vi "MGI Set Z Scale Colors.vi"(7 "Scheme":T1=enum."Color Normal", 8 "error in (no error)":errorcluster, 9 "Min":dbl, 10 "Max":dbl, 11 "Scale or Intensity Graph Ref":refnum<vi>) -> (0 "error out":errorcluster, 2 "ValueScale":cluster{"Value":dbl, "Color":u32}[](array[cluster]) {"Value" format="%.1e"}, 3 "Ref (Duplicate)":refnum<vi>)   [LabVIEW 2020]
doc: "Updates the specified color scale using a distribution of colors specified by \"Scheme\". Min and Max describe the range of data that is to be displayed using the color scale.\nIf \"Z Scale Ref\" is not wired, the scale will not be updated but \"ValueScale\" will still contain data for the specified scheme.\nThe output \"ValueScale\" will have 256 color/data pairs.\n\nFreeware from Moore Good Ideas, Inc. www.MooreGoodIdeas.com\nDo not remove this line."
uses:
  <userlib>/_MGI/Graph/MGI Scale Color Scheme Enum.ctl
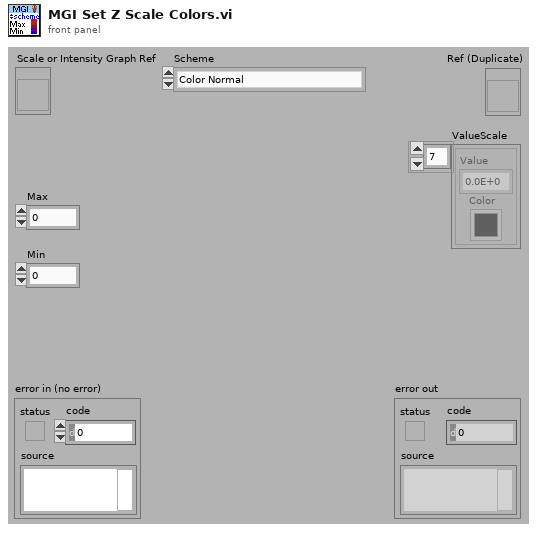
[diagram p1: front panel]
types:
  T1 = typedef "MGI Scale Color Scheme Enum.ctl" = enum16{"Gray Normal", "Gray Normal +-", "Gray Low", "Gray Low +-", "Gray High", "Gray High +-", "Gray Capped", "Color Normal", "Color Normal +-", "Color Low", "Color Low +-", "Color High", "Color High +-", "Color Cyclic", "Red White and Blue", "Red and Blue", "Black and White", "GrayN", "GrayN+-", "GrayL", "GrayL+-", "GrayH", "GrayH+-", "GrayC", "GrayAB", "BGRN", "BGRN+-", "BGRL", "BGRL+-", "BGRH", "BGRH+-", "Phase", "BGRAB", "BWR", "BR", "BkW"}
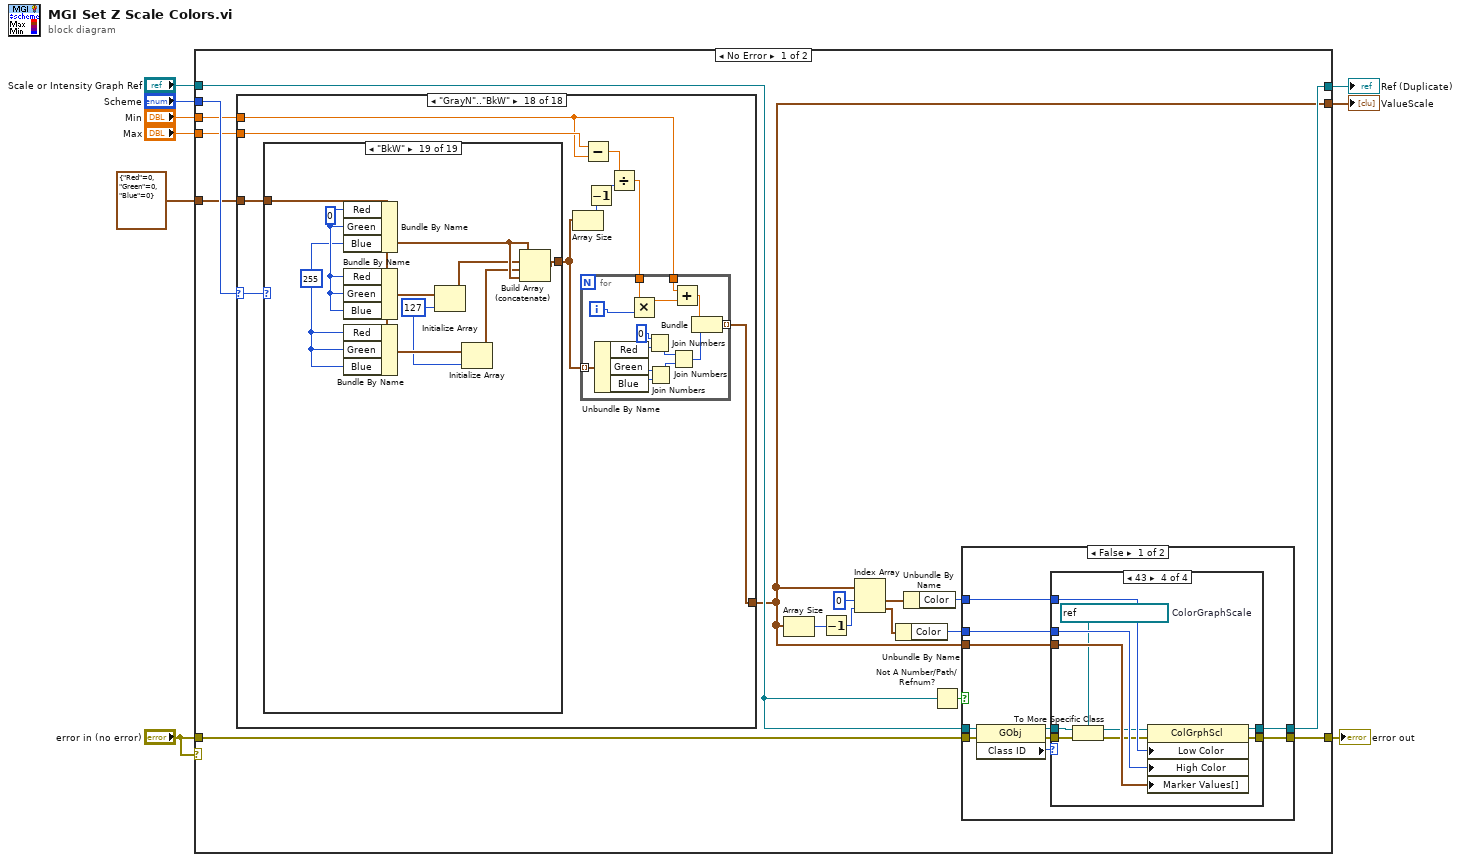
[diagram p0: block diagram]
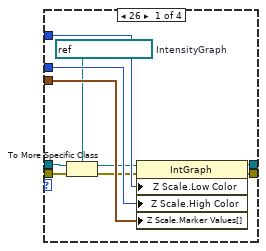
[diagram p2: hidden frame]
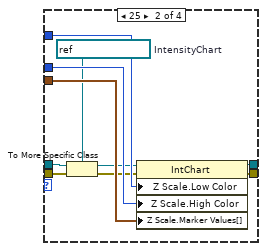
[diagram p3: hidden frame]
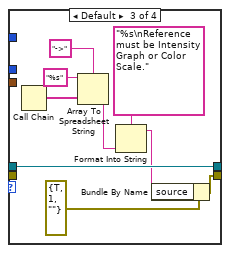
[diagram p4: hidden frame]
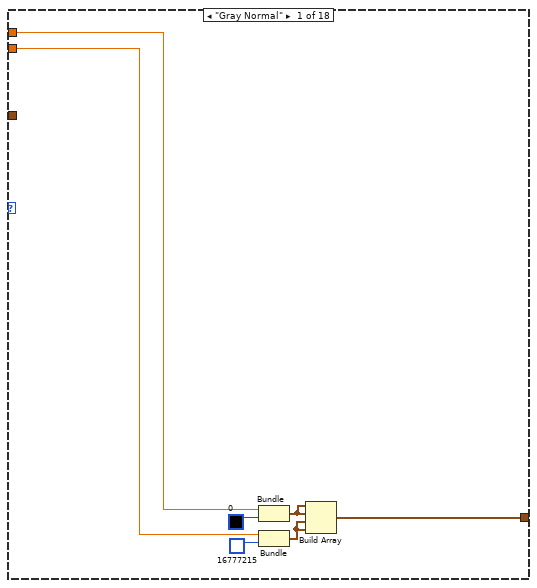
[diagram p6: hidden frame]
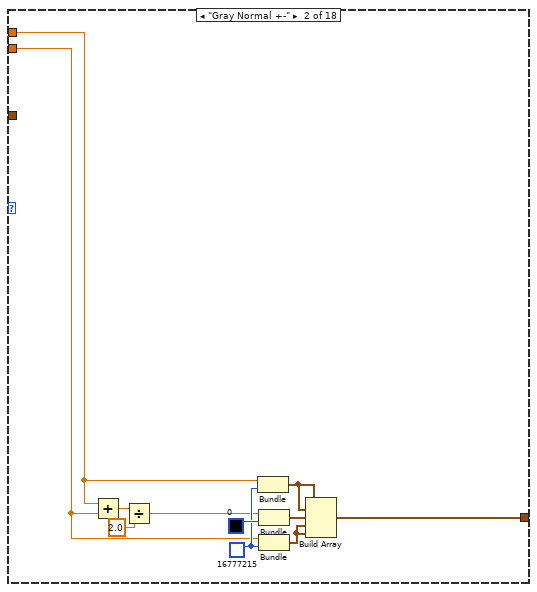
[diagram p7: hidden frame]
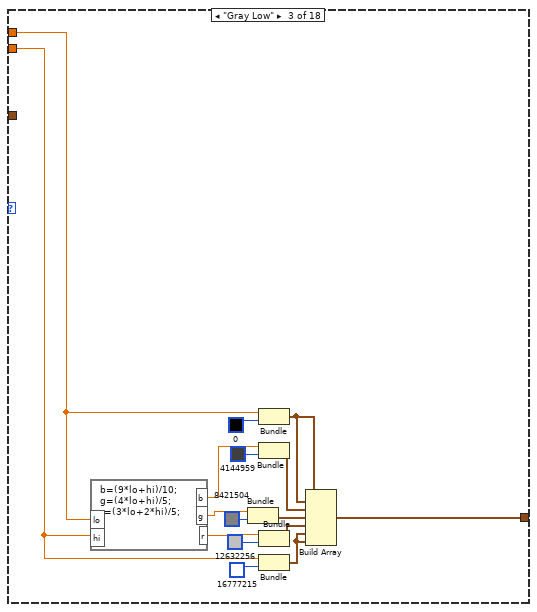
[diagram p8: hidden frame]
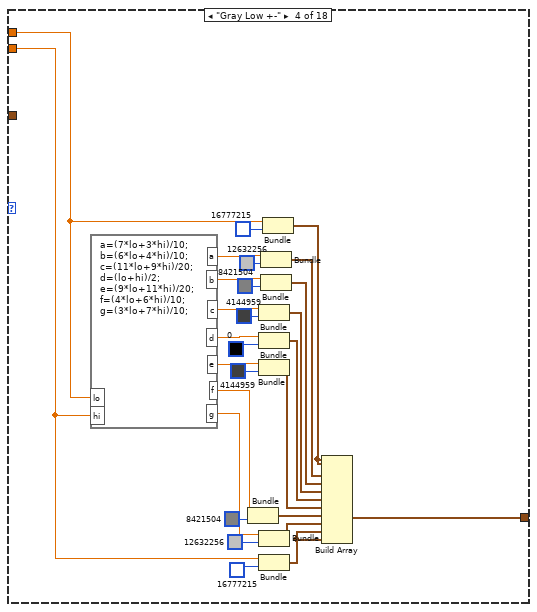
[diagram p9: hidden frame]
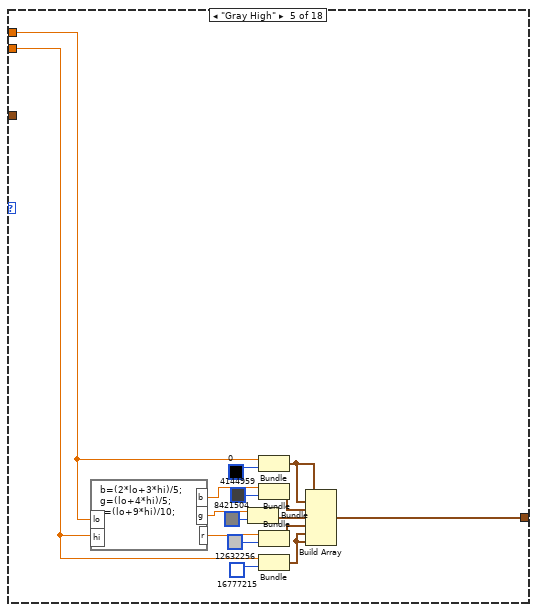
[diagram p10: hidden frame]
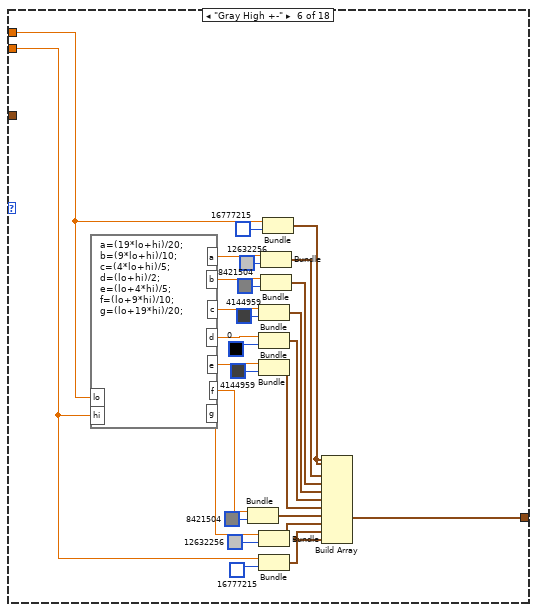
[diagram p11: hidden frame]
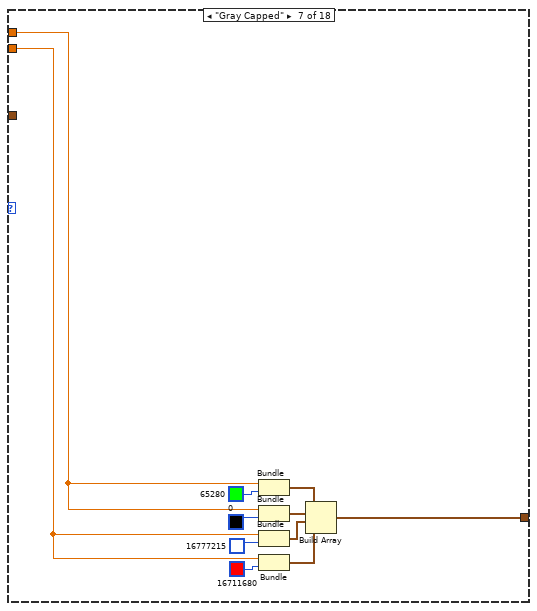
[diagram p12: hidden frame]
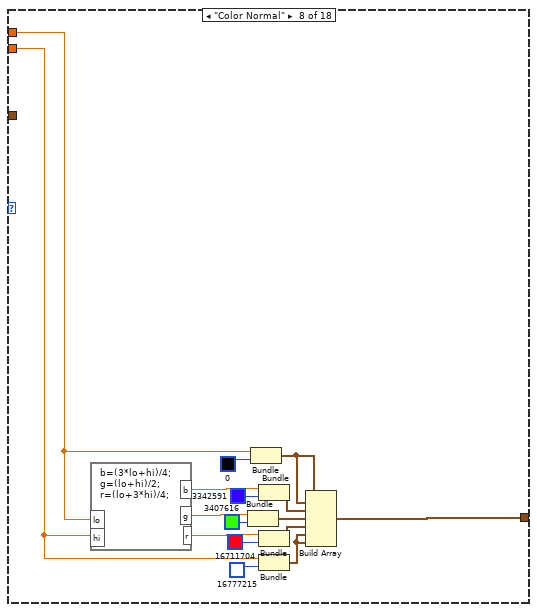
[diagram p13: hidden frame]
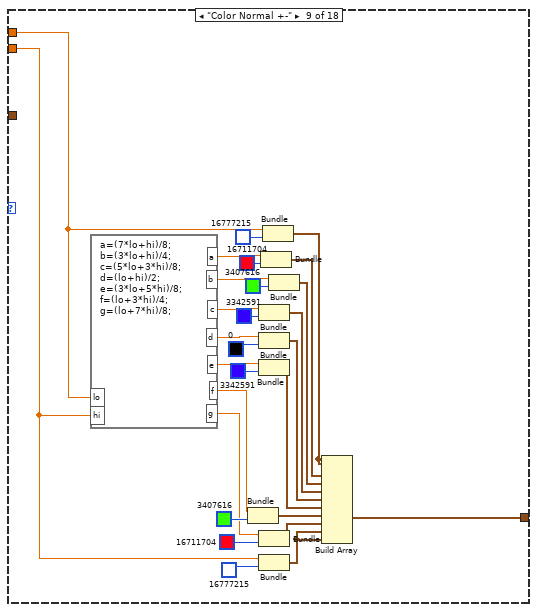
[diagram p14: hidden frame]
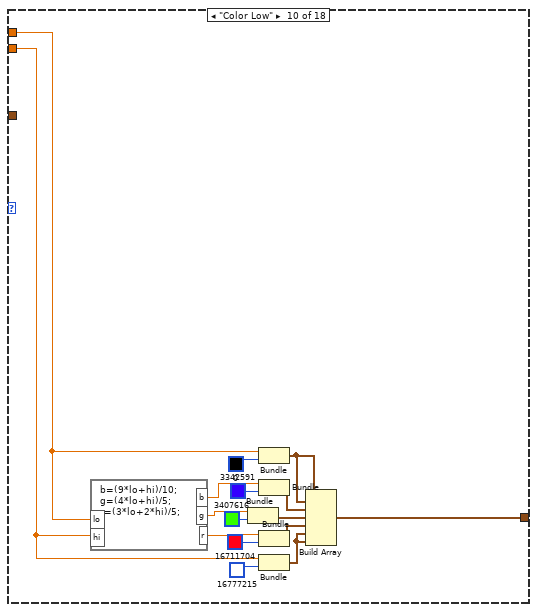
[diagram p15: hidden frame]
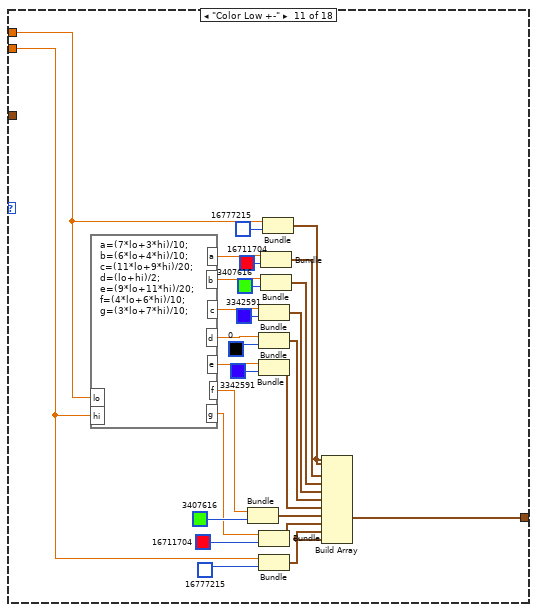
[diagram p16: hidden frame]
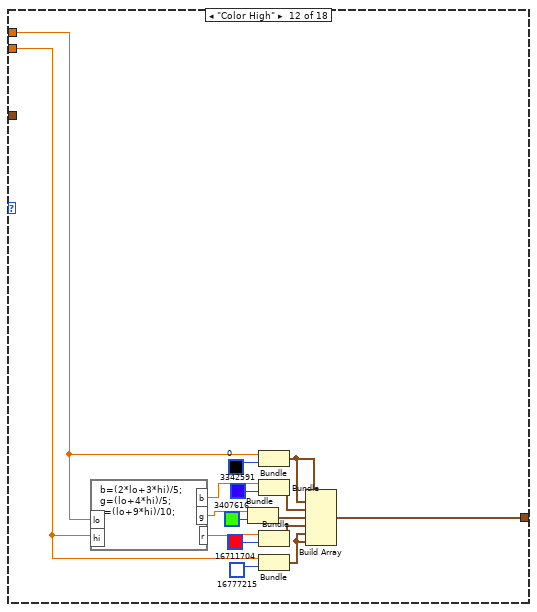
[diagram p17: hidden frame]
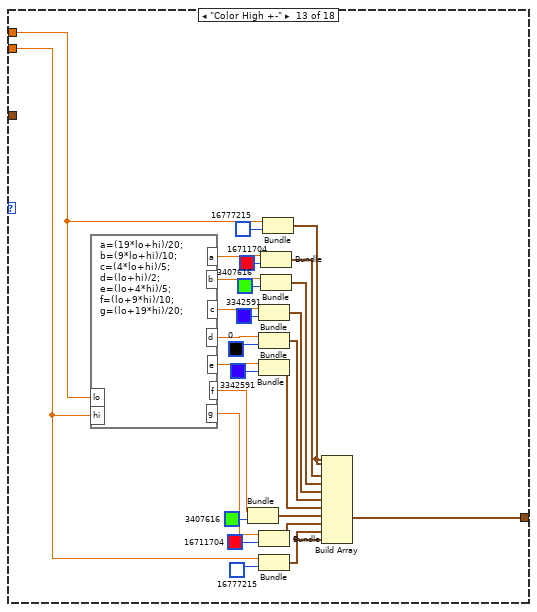
[diagram p18: hidden frame]
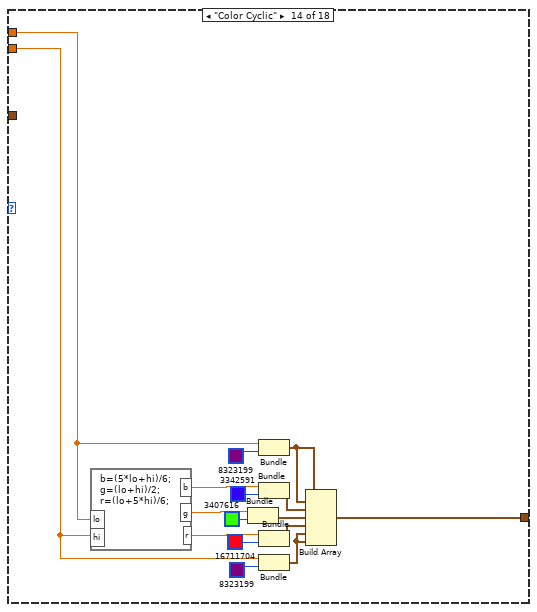
[diagram p19: hidden frame]
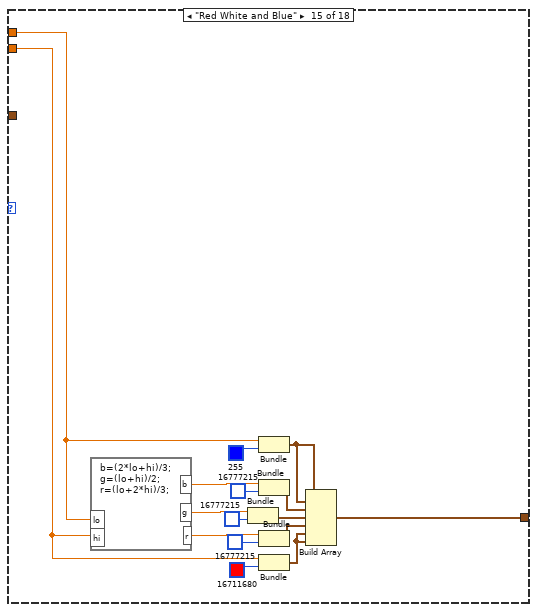
[diagram p20: hidden frame]
diagram:
  n1 = case shown="No Error" "error in (no error)" {
    tunnel: "Scheme" -> [w26 _]
    tunnel: "Min" -> [w25 _]
    tunnel: "Max" -> [w24 _]
    tunnel: [w23 w940] -> w6
    tunnel: "error in (no error)" -> [w22 w941]
    tunnel: [w21 w941] -> w5
    tunnel: [w11 _] -> w4
    tunnel: "Scale or Intensity Graph Ref" -> [w13 w940]
    tunnel: cluster{"Red":u8, "Green":u8, "Blue":u8} {"Red"=0, "Green"=0, "Blue"=0} ("Color Value") -> [w10 _]
    frame No Error {
      n2 = case shown="\"GrayN\"..\"BkW\"" w26 {
        selector: w26 -> [_ _ _ _ _ _ _ _ _ _ _ _ _ _ _ _ _ w400]
        tunnel: w25 -> [w81 w90 w99 w124 w143 w168 w187 w198 w223 w242 w267 w286 w311 w327 w346 w362 w378 w397]
        tunnel: w24 -> [w80 w89 w98 w127 w142 w171 w185 w197 w226 w241 w270 w285 w314 w330 w345 w360 w377 w398]
        tunnel: [w84 w95 w111 w139 w155 w183 w194 w210 w238 w254 w282 w298 w326 w342 w358 w374 w390 w391] -> w11
        tunnel: w10 -> [_ _ _ _ _ _ _ _ _ _ _ _ _ _ _ _ _ w399]
        frame "Gray Normal" {
          n3 = Bundle("Min"=w81, "Color"=u32 0) -> (w78:cluster{"Min":dbl, "Color":u32})  [unwired: 1 out]
          n4 = Bundle("Max"=w80, "Color"=u32 16777215) -> (w79:cluster{"Max":dbl, "Color":u32})  [unwired: 1 out]
          n5 = Build Array(w78, w78, w79, w79) -> (w84:cluster{"Max":dbl, "Color":u32}[])
        }
        frame "Gray Normal +-" {
          w91 = u32 16777215 ("Color")
          n6 = Add(x=w90, y=w89) -> (x+y=w88:dbl)
          n7 = Divide(x=w88, y=2.0) -> (x/y=w86:dbl)
          n8 = Bundle("Min"=w90, "Color"=w91) -> (w85:cluster{"Min":dbl, "Color":u32})  [unwired: 1 out]
          n9 = Bundle(w86, "Color"=u32 0) -> (w92:cluster{dbl, "Color":u32})  [unwired: 1 out]
          n10 = Bundle("Max"=w89, "Color"=w91) -> (w93:cluster{"Max":dbl, "Color":u32})  [unwired: 1 out]
          n11 = Build Array(w85, w85, w92, w93, w93) -> (w95:cluster{"Max":dbl, "Color":u32}[])
        }
        frame "Gray Low" {
          n12 = formula code="b=(9*lo+hi)/10;\ng=(4*lo+hi)/5;\nr=(3*lo+2*hi)/5;"("lo"=w99, "hi"=w98) -> ("b"=w105:dbl, "g"=w106:dbl, "r"=w107:dbl)
          n13 = Bundle("g"=w106, "Color"=u32 8421504) -> (w103:cluster{"g":dbl, "Color":u32})  [unwired: 1 out]
          n14 = Bundle("Min"=w99, "Color"=u32 0) -> (w96:cluster{"Min":dbl, "Color":u32})  [unwired: 1 out]
          n15 = Bundle("b"=w105, "Color"=u32 4144959) -> (w104:cluster{"b":dbl, "Color":u32})  [unwired: 1 out]
          n16 = Bundle("r"=w107, "Color"=u32 12632256) -> (w102:cluster{"r":dbl, "Color":u32})  [unwired: 1 out]
          n17 = Bundle("Max"=w98, "Color"=u32 16777215) -> (w97:cluster{"Max":dbl, "Color":u32})  [unwired: 1 out]
          n18 = Build Array(w96, w96, w104, w103, w102, w97, w97) -> (w111:cluster{"Max":dbl, "Color":u32}[])
        }
        frame "Gray Low +-" {
          n19 = formula code="a=(7*lo+3*hi)/10;\nb=(6*lo+4*hi)/10;\nc=(11*lo+9*hi)/20;\nd=(lo+hi)/2;\ne=(9*lo+11*hi)/20;\nf=(4*lo+6*hi)/10;\ng=(3*lo+7*hi)/10;"("lo"=w124, "hi"=w127) -> ("e"=w133:dbl, "f"=w134:dbl, "g"=w135:dbl, "a"=w115:dbl, "b"=w114:dbl, "c"=w113:dbl, "d"=w112:dbl)
          n20 = Bundle("f"=w134, "Color"=u32 8421504) -> (w131:cluster{"f":dbl, "Color":u32})  [unwired: 1 out]
          n21 = Bundle("c"=w113, "Color"=u32 4144959) -> (w118:cluster{"c":dbl, "Color":u32})  [unwired: 1 out]
          n22 = Bundle("d"=w112, "Color"=u32 0) -> (w125:cluster{"d":dbl, "Color":u32})  [unwired: 1 out]
          n23 = Bundle("e"=w133, "Color"=u32 4144959) -> (w132:cluster{"e":dbl, "Color":u32})  [unwired: 1 out]
          n24 = Bundle("g"=w135, "Color"=u32 12632256) -> (w130:cluster{"g":dbl, "Color":u32})  [unwired: 1 out]
          n25 = Bundle("Max"=w127, "Color"=u32 16777215) -> (w126:cluster{"Max":dbl, "Color":u32})  [unwired: 1 out]
          n26 = Bundle("a"=w115, "Color"=u32 12632256) -> (w116:cluster{"a":dbl, "Color":u32})  [unwired: 1 out]
          n27 = Bundle("b"=w114, "Color"=u32 8421504) -> (w117:cluster{"b":dbl, "Color":u32})  [unwired: 1 out]
          n28 = Bundle("Min"=w124, "Color"=u32 16777215) -> (w123:cluster{"Min":dbl, "Color":u32})  [unwired: 1 out]
          n29 = Build Array(w123, w123, w116, w117, w118, w125, w132, w131, w130, w126, w126) -> (w139:cluster{"Max":dbl, "Color":u32}[])
        }
        frame "Gray High" {
          n30 = formula code="b=(2*lo+3*hi)/5;\ng=(lo+4*hi)/5;\nr=(lo+9*hi)/10;"("lo"=w143, "hi"=w142) -> ("b"=w149:dbl, "g"=w150:dbl, "r"=w151:dbl)
          n31 = Bundle("g"=w150, "Color"=u32 8421504) -> (w147:cluster{"g":dbl, "Color":u32})  [unwired: 1 out]
          n32 = Bundle("Min"=w143, "Color"=u32 0) -> (w141:cluster{"Min":dbl, "Color":u32})  [unwired: 1 out]
          n33 = Bundle("b"=w149, "Color"=u32 4144959) -> (w148:cluster{"b":dbl, "Color":u32})  [unwired: 1 out]
          n34 = Bundle("r"=w151, "Color"=u32 12632256) -> (w146:cluster{"r":dbl, "Color":u32})  [unwired: 1 out]
          n35 = Bundle("Max"=w142, "Color"=u32 16777215) -> (w140:cluster{"Max":dbl, "Color":u32})  [unwired: 1 out]
          n36 = Build Array(w141, w141, w148, w147, w146, w140, w140) -> (w155:cluster{"Max":dbl, "Color":u32}[])
        }
        frame "Gray High +-" {
          n37 = formula code="a=(19*lo+hi)/20;\nb=(9*lo+hi)/10;\nc=(4*lo+hi)/5;\nd=(lo+hi)/2;\ne=(lo+4*hi)/5;\nf=(lo+9*hi)/10;\ng=(lo+19*hi)/20;"("lo"=w168, "hi"=w171) -> ("e"=w177:dbl, "f"=w178:dbl, "g"=w179:dbl, "a"=w159:dbl, "b"=w158:dbl, "c"=w157:dbl, "d"=w156:dbl)
          n38 = Bundle("f"=w178, "Color"=u32 8421504) -> (w175:cluster{"f":dbl, "Color":u32})  [unwired: 1 out]
          n39 = Bundle("c"=w157, "Color"=u32 4144959) -> (w162:cluster{"c":dbl, "Color":u32})  [unwired: 1 out]
          n40 = Bundle("d"=w156, "Color"=u32 0) -> (w169:cluster{"d":dbl, "Color":u32})  [unwired: 1 out]
          n41 = Bundle("e"=w177, "Color"=u32 4144959) -> (w176:cluster{"e":dbl, "Color":u32})  [unwired: 1 out]
          n42 = Bundle("g"=w179, "Color"=u32 12632256) -> (w174:cluster{"g":dbl, "Color":u32})  [unwired: 1 out]
          n43 = Bundle("Max"=w171, "Color"=u32 16777215) -> (w170:cluster{"Max":dbl, "Color":u32})  [unwired: 1 out]
          n44 = Bundle("a"=w159, "Color"=u32 12632256) -> (w160:cluster{"a":dbl, "Color":u32})  [unwired: 1 out]
          n45 = Bundle("b"=w158, "Color"=u32 8421504) -> (w161:cluster{"b":dbl, "Color":u32})  [unwired: 1 out]
          n46 = Bundle("Min"=w168, "Color"=u32 16777215) -> (w167:cluster{"Min":dbl, "Color":u32})  [unwired: 1 out]
          n47 = Build Array(w167, w167, w160, w161, w162, w169, w176, w175, w174, w170, w170) -> (w183:cluster{"Max":dbl, "Color":u32}[])
        }
        frame "Gray Capped" {
          n48 = Bundle("Min"=w187, "Color"=u32 65280) -> (w186:cluster{"Min":dbl, "Color":u32})  [unwired: 1 out]
          n49 = Bundle("Min"=w187, "Color"=u32 0) -> (w192:cluster{"Min":dbl, "Color":u32})  [unwired: 1 out]
          n50 = Bundle("Max"=w185, "Color"=u32 16777215) -> (w193:cluster{"Max":dbl, "Color":u32})  [unwired: 1 out]
          n51 = Bundle("Max"=w185, "Color"=u32 16711680) -> (w184:cluster{"Max":dbl, "Color":u32})  [unwired: 1 out]
          n52 = Build Array(w186, w192, w193, w184) -> (w194:cluster{"Max":dbl, "Color":u32}[])
        }
        frame "Color Normal" {
          n53 = formula code="b=(3*lo+hi)/4;\ng=(lo+hi)/2;\nr=(lo+3*hi)/4;"("lo"=w198, "hi"=w197) -> ("b"=w204:dbl, "g"=w205:dbl, "r"=w206:dbl)
          n54 = Bundle("g"=w205, "Color"=u32 3407616) -> (w202:cluster{"g":dbl, "Color":u32})  [unwired: 1 out]
          n55 = Bundle("Min"=w198, "Color"=u32 0) -> (w195:cluster{"Min":dbl, "Color":u32})  [unwired: 1 out]
          n56 = Bundle("b"=w204, "Color"=u32 3342591) -> (w203:cluster{"b":dbl, "Color":u32})  [unwired: 1 out]
          n57 = Bundle("r"=w206, "Color"=u32 16711704) -> (w201:cluster{"r":dbl, "Color":u32})  [unwired: 1 out]
          n58 = Bundle("Max"=w197, "Color"=u32 16777215) -> (w196:cluster{"Max":dbl, "Color":u32})  [unwired: 1 out]
          n59 = Build Array(w195, w195, w203, w202, w201, w196, w196) -> (w210:cluster{"Max":dbl, "Color":u32}[])
        }
        frame "Color Normal +-" {
          n60 = formula code="a=(7*lo+hi)/8;\nb=(3*lo+hi)/4;\nc=(5*lo+3*hi)/8;\nd=(lo+hi)/2;\ne=(3*lo+5*hi)/8;\nf=(lo+3*hi)/4;\ng=(lo+7*hi)/8;"("lo"=w223, "hi"=w226) -> ("e"=w232:dbl, "f"=w233:dbl, "g"=w234:dbl, "a"=w214:dbl, "b"=w213:dbl, "c"=w212:dbl, "d"=w211:dbl)
          n61 = Bundle("f"=w233, "Color"=u32 3407616) -> (w230:cluster{"f":dbl, "Color":u32})  [unwired: 1 out]
          n62 = Bundle("c"=w212, "Color"=u32 3342591) -> (w217:cluster{"c":dbl, "Color":u32})  [unwired: 1 out]
          n63 = Bundle("d"=w211, "Color"=u32 0) -> (w224:cluster{"d":dbl, "Color":u32})  [unwired: 1 out]
          n64 = Bundle("e"=w232, "Color"=u32 3342591) -> (w231:cluster{"e":dbl, "Color":u32})  [unwired: 1 out]
          n65 = Bundle("g"=w234, "Color"=u32 16711704) -> (w229:cluster{"g":dbl, "Color":u32})  [unwired: 1 out]
          n66 = Bundle("Max"=w226, "Color"=u32 16777215) -> (w225:cluster{"Max":dbl, "Color":u32})  [unwired: 1 out]
          n67 = Bundle("a"=w214, "Color"=u32 16711704) -> (w215:cluster{"a":dbl, "Color":u32})  [unwired: 1 out]
          n68 = Bundle("Min"=w223, "Color"=u32 16777215) -> (w222:cluster{"Min":dbl, "Color":u32})  [unwired: 1 out]
          n69 = Bundle("b"=w213, "Color"=u32 3407616) -> (w216:cluster{"b":dbl, "Color":u32})  [unwired: 1 out]
          n70 = Build Array(w222, w222, w215, w216, w217, w224, w231, w230, w229, w225, w225) -> (w238:cluster{"Max":dbl, "Color":u32}[])
        }
        frame "Color Low" {
          n71 = formula code="b=(9*lo+hi)/10;\ng=(4*lo+hi)/5;\nr=(3*lo+2*hi)/5;"("lo"=w242, "hi"=w241) -> ("b"=w248:dbl, "g"=w249:dbl, "r"=w250:dbl)
          n72 = Bundle("g"=w249, "Color"=u32 3407616) -> (w246:cluster{"g":dbl, "Color":u32})  [unwired: 1 out]
          n73 = Bundle("Min"=w242, "Color"=u32 0) -> (w239:cluster{"Min":dbl, "Color":u32})  [unwired: 1 out]
          n74 = Bundle("b"=w248, "Color"=u32 3342591) -> (w247:cluster{"b":dbl, "Color":u32})  [unwired: 1 out]
          n75 = Bundle("r"=w250, "Color"=u32 16711704) -> (w245:cluster{"r":dbl, "Color":u32})  [unwired: 1 out]
          n76 = Bundle("Max"=w241, "Color"=u32 16777215) -> (w240:cluster{"Max":dbl, "Color":u32})  [unwired: 1 out]
          n77 = Build Array(w239, w239, w247, w246, w245, w240, w240) -> (w254:cluster{"Max":dbl, "Color":u32}[])
        }
        frame "Color Low +-" {
          n78 = formula code="a=(7*lo+3*hi)/10;\nb=(6*lo+4*hi)/10;\nc=(11*lo+9*hi)/20;\nd=(lo+hi)/2;\ne=(9*lo+11*hi)/20;\nf=(4*lo+6*hi)/10;\ng=(3*lo+7*hi)/10;"("lo"=w267, "hi"=w270) -> ("e"=w276:dbl, "f"=w277:dbl, "g"=w278:dbl, "a"=w258:dbl, "b"=w257:dbl, "c"=w256:dbl, "d"=w255:dbl)
          n79 = Bundle("f"=w277, "Color"=u32 3407616) -> (w274:cluster{"f":dbl, "Color":u32})  [unwired: 1 out]
          n80 = Bundle("c"=w256, "Color"=u32 3342591) -> (w261:cluster{"c":dbl, "Color":u32})  [unwired: 1 out]
          n81 = Bundle("d"=w255, "Color"=u32 0) -> (w268:cluster{"d":dbl, "Color":u32})  [unwired: 1 out]
          n82 = Bundle("e"=w276, "Color"=u32 3342591) -> (w275:cluster{"e":dbl, "Color":u32})  [unwired: 1 out]
          n83 = Bundle("g"=w278, "Color"=u32 16711704) -> (w273:cluster{"g":dbl, "Color":u32})  [unwired: 1 out]
          n84 = Bundle("Max"=w270, "Color"=u32 16777215) -> (w269:cluster{"Max":dbl, "Color":u32})  [unwired: 1 out]
          n85 = Bundle("a"=w258, "Color"=u32 16711704) -> (w259:cluster{"a":dbl, "Color":u32})  [unwired: 1 out]
          n86 = Bundle("b"=w257, "Color"=u32 3407616) -> (w260:cluster{"b":dbl, "Color":u32})  [unwired: 1 out]
          n87 = Bundle("Min"=w267, "Color"=u32 16777215) -> (w266:cluster{"Min":dbl, "Color":u32})  [unwired: 1 out]
          n88 = Build Array(w266, w266, w259, w260, w261, w268, w275, w274, w273, w269, w269) -> (w282:cluster{"Max":dbl, "Color":u32}[])
        }
        frame "Color High" {
          n89 = formula code="b=(2*lo+3*hi)/5;\ng=(lo+4*hi)/5;\nr=(lo+9*hi)/10;"("lo"=w286, "hi"=w285) -> ("b"=w292:dbl, "g"=w293:dbl, "r"=w294:dbl)
          n90 = Bundle("g"=w293, "Color"=u32 3407616) -> (w290:cluster{"g":dbl, "Color":u32})  [unwired: 1 out]
          n91 = Bundle("Min"=w286, "Color"=u32 0) -> (w283:cluster{"Min":dbl, "Color":u32})  [unwired: 1 out]
          n92 = Bundle("b"=w292, "Color"=u32 3342591) -> (w291:cluster{"b":dbl, "Color":u32})  [unwired: 1 out]
          n93 = Bundle("r"=w294, "Color"=u32 16711704) -> (w289:cluster{"r":dbl, "Color":u32})  [unwired: 1 out]
          n94 = Bundle("Max"=w285, "Color"=u32 16777215) -> (w284:cluster{"Max":dbl, "Color":u32})  [unwired: 1 out]
          n95 = Build Array(w283, w283, w291, w290, w289, w284, w284) -> (w298:cluster{"Max":dbl, "Color":u32}[])
        }
        frame "Color High +-" {
          n96 = formula code="a=(19*lo+hi)/20;\nb=(9*lo+hi)/10;\nc=(4*lo+hi)/5;\nd=(lo+hi)/2;\ne=(lo+4*hi)/5;\nf=(lo+9*hi)/10;\ng=(lo+19*hi)/20;"("lo"=w311, "hi"=w314) -> ("e"=w320:dbl, "f"=w321:dbl, "g"=w322:dbl, "a"=w302:dbl, "b"=w301:dbl, "c"=w300:dbl, "d"=w299:dbl)
          n97 = Bundle("f"=w321, "Color"=u32 3407616) -> (w318:cluster{"f":dbl, "Color":u32})  [unwired: 1 out]
          n98 = Bundle("c"=w300, "Color"=u32 3342591) -> (w305:cluster{"c":dbl, "Color":u32})  [unwired: 1 out]
          n99 = Bundle("d"=w299, "Color"=u32 0) -> (w312:cluster{"d":dbl, "Color":u32})  [unwired: 1 out]
          n100 = Bundle("e"=w320, "Color"=u32 3342591) -> (w319:cluster{"e":dbl, "Color":u32})  [unwired: 1 out]
          n101 = Bundle("g"=w322, "Color"=u32 16711704) -> (w317:cluster{"g":dbl, "Color":u32})  [unwired: 1 out]
          n102 = Bundle("Max"=w314, "Color"=u32 16777215) -> (w313:cluster{"Max":dbl, "Color":u32})  [unwired: 1 out]
          n103 = Bundle("a"=w302, "Color"=u32 16711704) -> (w303:cluster{"a":dbl, "Color":u32})  [unwired: 1 out]
          n104 = Bundle("b"=w301, "Color"=u32 3407616) -> (w304:cluster{"b":dbl, "Color":u32})  [unwired: 1 out]
          n105 = Bundle("Min"=w311, "Color"=u32 16777215) -> (w310:cluster{"Min":dbl, "Color":u32})  [unwired: 1 out]
          n106 = Build Array(w310, w310, w303, w304, w305, w312, w319, w318, w317, w313, w313) -> (w326:cluster{"Max":dbl, "Color":u32}[])
        }
        frame "Color Cyclic" {
          n107 = formula code="b=(5*lo+hi)/6;\ng=(lo+hi)/2;\nr=(lo+5*hi)/6;"("lo"=w327, "hi"=w330) -> ("b"=w336:dbl, "g"=w337:dbl, "r"=w338:dbl)
          n108 = Bundle("g"=w337, "Color"=u32 3407616) -> (w334:cluster{"g":dbl, "Color":u32})  [unwired: 1 out]
          n109 = Bundle("Min"=w327, "Color"=u32 8323199) -> (w328:cluster{"Min":dbl, "Color":u32})  [unwired: 1 out]
          n110 = Bundle("b"=w336, "Color"=u32 3342591) -> (w335:cluster{"b":dbl, "Color":u32})  [unwired: 1 out]
          n111 = Bundle("r"=w338, "Color"=u32 16711704) -> (w333:cluster{"r":dbl, "Color":u32})  [unwired: 1 out]
          n112 = Bundle("Max"=w330, "Color"=u32 8323199) -> (w329:cluster{"Max":dbl, "Color":u32})  [unwired: 1 out]
          n113 = Build Array(w328, w328, w335, w334, w333, w329, w329) -> (w342:cluster{"Max":dbl, "Color":u32}[])
        }
        frame "Red White and Blue" {
          n114 = formula code="b=(2*lo+hi)/3;\ng=(lo+hi)/2;\nr=(lo+2*hi)/3;"("lo"=w346, "hi"=w345) -> ("b"=w352:dbl, "g"=w353:dbl, "r"=w354:dbl)
          n115 = Bundle("g"=w353, "Color"=u32 16777215) -> (w350:cluster{"g":dbl, "Color":u32})  [unwired: 1 out]
          n116 = Bundle("Min"=w346, "Color"=u32 255) -> (w343:cluster{"Min":dbl, "Color":u32})  [unwired: 1 out]
          n117 = Bundle("b"=w352, "Color"=u32 16777215) -> (w351:cluster{"b":dbl, "Color":u32})  [unwired: 1 out]
          n118 = Bundle("r"=w354, "Color"=u32 16777215) -> (w349:cluster{"r":dbl, "Color":u32})  [unwired: 1 out]
          n119 = Bundle("Max"=w345, "Color"=u32 16711680) -> (w344:cluster{"Max":dbl, "Color":u32})  [unwired: 1 out]
          n120 = Build Array(w343, w343, w351, w350, w349, w344, w344) -> (w358:cluster{"Max":dbl, "Color":u32}[])
        }
        frame "Red and Blue" {
          w363 = u32 16711680 ("Color")
          w364 = u32 255 ("Color")
          n121 = Add(x=w362, y=w360) -> (x+y=w370:dbl)
          n122 = Divide(x=w370, y=2.0) -> (x/y=w367:dbl)
          n123 = Bundle(w367, "Color"=u32 12566527) -> (w365:cluster{dbl, "Color":u32})  [unwired: 1 out]
          n124 = Bundle(w367, "Color"=u32 16760767) -> (w366:cluster{dbl, "Color":u32})  [unwired: 1 out]
          n125 = Bundle("Min"=w362, "Color"=w364) -> (w361:cluster{"Min":dbl, "Color":u32})  [unwired: 1 out]
          n126 = Bundle("Min"=w362, "Color"=w364) -> (w372:cluster{"Min":dbl, "Color":u32})  [unwired: 1 out]
          n127 = Bundle("Max"=w360, "Color"=w363) -> (w373:cluster{"Max":dbl, "Color":u32})  [unwired: 1 out]
          n128 = Bundle("Max"=w360, "Color"=w363) -> (w359:cluster{"Max":dbl, "Color":u32})  [unwired: 1 out]
          n129 = Build Array(w361, w372, w365, w366, w373, w359) -> (w374:cluster{"Max":dbl, "Color":u32}[])
        }
        frame "Black and White" {
          w382 = u32 16777215 ("Color")
          w385 = u32 0 ("Color")
          n130 = Add(x=w378, y=w377) -> (x+y=w384:dbl)
          n131 = Divide(x=w384, y=2.0) -> (x/y=w381:dbl)
          n132 = Bundle(w381, "Color"=w385) -> (w379:cluster{dbl, "Color":u32})  [unwired: 1 out]
          n133 = Bundle(w381, "Color"=w382) -> (w380:cluster{dbl, "Color":u32})  [unwired: 1 out]
          n134 = Bundle("Min"=w378, "Color"=u32 16860) -> (w375:cluster{"Min":dbl, "Color":u32})  [unwired: 1 out]
          n135 = Bundle("Min"=w378, "Color"=w385) -> (w388:cluster{"Min":dbl, "Color":u32})  [unwired: 1 out]
          n136 = Bundle("Max"=w377, "Color"=w382) -> (w389:cluster{"Max":dbl, "Color":u32})  [unwired: 1 out]
          n137 = Bundle("Max"=w377, "Color"=u32 16860) -> (w376:cluster{"Max":dbl, "Color":u32})  [unwired: 1 out]
          n138 = Build Array(w375, w388, w379, w380, w389, w376) -> (w390:cluster{"Max":dbl, "Color":u32}[])
        }
        frame "GrayN".."BkW" {
          n139 = case shown="\"BkW\"" w400 {
            tunnel: [w415 w423 w430 w456 w482 w504 w528 w542 w558 w599 w639 w682 w720 w765 w803 w848 w893 w914 w939] -> w395
            tunnel: w399 -> [w416 w424 w436 w462 w486 w512 w534 w548 w561 w598 w644 w685 w727 w768 w811 w849 w894 w913 w938]
            frame "Gray Normal".."GrayN" {
              n140 = for {
                N: 256 -> [_]
                tunnel: w416 -> [w420]
                tunnel: [w418] -> w415 mode=indexing
                i -> [w419]
                n141 = Bundle By Name(cluster=w420, "Red"=w419, "Green"=w419, "Blue"=w419) -> (w418:cluster{"Red":u8, "Green":u8, "Blue":u8})
              }
            }
            frame "GrayN+-" {
              n142 = for {
                N: 128 -> [_]
                tunnel: w424 -> [w429]
                tunnel: [w428] -> w422 mode=indexing
                i -> [w426]
                n143 = Add(x=w426, y=w426) -> (x+y=w427:i32)
                n144 = Bundle By Name(cluster=w429, "Red"=w427, "Green"=w427, "Blue"=w427) -> (w428:cluster{"Red":u8, "Green":u8, "Blue":u8})
              }
              n145 = Reverse 1D Array(array=w422) -> (reversed array=w421:cluster{"Red":u8, "Green":u8, "Blue":u8}[])
              n146 = Build Array (concatenate)(w421, w422) -> (w423:cluster{"Red":u8, "Green":u8, "Blue":u8}[])
            }
            frame "GrayL" {
              w438 = 64
              n147 = for {
                N: w438 -> [_]
                tunnel: w436 -> [w455]
                tunnel: [w451] -> w435 mode=indexing
                i -> [w454]
                n148 = Multiply(x=w454, y=2) -> (x*y=w452:i32)
                n149 = Bundle By Name(cluster=w455, "Red"=w452, "Green"=w452, "Blue"=w452) -> (w451:cluster{"Red":u8, "Green":u8, "Blue":u8})
              }
              n150 = for {
                N: w438 -> [_]
                tunnel: w436 -> [w450]
                tunnel: [w447] -> w433 mode=indexing
                i -> [w446]
                n151 = Add(x=w446, y=128) -> (x+y=w448:i32)
                n152 = Bundle By Name(cluster=w450, "Red"=w448, "Green"=w448, "Blue"=w448) -> (w447:cluster{"Red":u8, "Green":u8, "Blue":u8})
              }
              n153 = for {
                N: 128 -> [_]
                tunnel: w436 -> [w445]
                tunnel: [w444] -> w434 mode=indexing
                i -> [w441]
                n154 = Quotient & Remainder(x=w441, y=2) -> (floor(x/y)=w440:i32)  [unwired: 1 out]
                n155 = Add(x=192, y=w440) -> (x+y=w442:i32)
                n156 = Bundle By Name(cluster=w445, "Red"=w442, "Green"=w442, "Blue"=w442) -> (w444:cluster{"Red":u8, "Green":u8, "Blue":u8})
              }
              n157 = Build Array (concatenate)(w435, w433, w434) -> (w432:cluster{"Red":u8, "Green":u8, "Blue":u8}[])
              n158 = Reverse 1D Array(array=w432) -> (reversed array=w431:cluster{"Red":u8, "Green":u8, "Blue":u8}[])
              n159 = Build Array (concatenate)(w431, w432) -> (w430:cluster{"Red":u8, "Green":u8, "Blue":u8}[])
            }
            frame "GrayL+-" {
              w464 = 32
              n160 = for {
                N: w464 -> [_]
                tunnel: w462 -> [w479]
                tunnel: [w475] -> w461 mode=indexing
                i -> [w478]
                n161 = Multiply(x=w478, y=4) -> (x*y=w476:i32)
                n162 = Bundle By Name(cluster=w479, "Red"=w476, "Green"=w476, "Blue"=w476) -> (w475:cluster{"Red":u8, "Green":u8, "Blue":u8})
              }
              n163 = for {
                N: w464 -> [_]
                tunnel: w462 -> [w474]
                tunnel: [w471] -> w459 mode=indexing
                i -> [w470]
                n164 = Compound Arithmetic op=ADD(w470, w470, 128 ("y")) -> (w472:i32)
                n165 = Bundle By Name(cluster=w474, "Red"=w472, "Green"=w472, "Blue"=w472) -> (w471:cluster{"Red":u8, "Green":u8, "Blue":u8})
              }
              n166 = for {
                N: 64 -> [_]
                tunnel: w462 -> [w469]
                tunnel: [w468] -> w460 mode=indexing
                i -> [w465]
                n167 = Add(x=192, y=w465) -> (x+y=w466:i32)
                n168 = Bundle By Name(cluster=w469, "Red"=w466, "Green"=w466, "Blue"=w466) -> (w468:cluster{"Red":u8, "Green":u8, "Blue":u8})
              }
              n169 = Build Array (concatenate)(w461, w459, w460) -> (w458:cluster{"Red":u8, "Green":u8, "Blue":u8}[])
              n170 = Reverse 1D Array(array=w458) -> (reversed array=w457:cluster{"Red":u8, "Green":u8, "Blue":u8}[])
              n171 = Build Array (concatenate)(w457, w458) -> (w456:cluster{"Red":u8, "Green":u8, "Blue":u8}[])
            }
            frame "GrayH" {
              w480 = 64
              n172 = for {
                N: 128 -> [_]
                tunnel: w486 -> [w503]
                tunnel: [w499] -> w485 mode=indexing
                i -> [w502]
                n173 = Quotient & Remainder(x=w502, y=2) -> (floor(x/y)=w500:i32)  [unwired: 1 out]
                n174 = Bundle By Name(cluster=w503, "Red"=w500, "Green"=w500, "Blue"=w500) -> (w499:cluster{"Red":u8, "Green":u8, "Blue":u8})
              }
              n175 = for {
                N: w480 -> [_]
                tunnel: w486 -> [w498]
                tunnel: [w494] -> w483 mode=indexing
                i -> [w497]
                n176 = Add(x=w497, y=64) -> (x+y=w495:i32)
                n177 = Bundle By Name(cluster=w498, "Red"=w495, "Green"=w495, "Blue"=w495) -> (w494:cluster{"Red":u8, "Green":u8, "Blue":u8})
              }
              n178 = for {
                N: w480 -> [_]
                tunnel: w486 -> [w493]
                tunnel: [w492] -> w484 mode=indexing
                i -> [w491]
                n179 = Multiply(x=w491, y=2) -> (x*y=w489:i32)
                n180 = Add(x=128, y=w489) -> (x+y=w487:i32)
                n181 = Bundle By Name(cluster=w493, "Red"=w487, "Green"=w487, "Blue"=w487) -> (w492:cluster{"Red":u8, "Green":u8, "Blue":u8})
              }
              n182 = Build Array (concatenate)(w485, w483, w484) -> (w482:cluster{"Red":u8, "Green":u8, "Blue":u8}[])
            }
            frame "GrayH+-" {
              w507 = 32
              n183 = for {
                N: 64 -> [_]
                tunnel: w512 -> [w527]
                tunnel: [w526] -> w511 mode=indexing
                i -> [w525]
                n184 = Bundle By Name(cluster=w527, "Red"=w525, "Green"=w525, "Blue"=w525) -> (w526:cluster{"Red":u8, "Green":u8, "Blue":u8})
              }
              n185 = for {
                N: w507 -> [_]
                tunnel: w512 -> [w524]
                tunnel: [w521] -> w509 mode=indexing
                i -> [w520]
                n186 = Compound Arithmetic op=ADD(w520, w520, 64 ("y")) -> (w522:i32)
                n187 = Bundle By Name(cluster=w524, "Red"=w522, "Green"=w522, "Blue"=w522) -> (w521:cluster{"Red":u8, "Green":u8, "Blue":u8})
              }
              n188 = for {
                N: w507 -> [_]
                tunnel: w512 -> [w519]
                tunnel: [w518] -> w510 mode=indexing
                i -> [w517]
                n189 = Multiply(x=w517, y=4) -> (x*y=w515:i32)
                n190 = Add(x=128, y=w515) -> (x+y=w513:i32)
                n191 = Bundle By Name(cluster=w519, "Red"=w513, "Green"=w513, "Blue"=w513) -> (w518:cluster{"Red":u8, "Green":u8, "Blue":u8})
              }
              n192 = Build Array (concatenate)(w511, w509, w510) -> (w506:cluster{"Red":u8, "Green":u8, "Blue":u8}[])
              n193 = Reverse 1D Array(array=w506) -> (reversed array=w505:cluster{"Red":u8, "Green":u8, "Blue":u8}[])
              n194 = Build Array (concatenate)(w505, w506) -> (w504:cluster{"Red":u8, "Green":u8, "Blue":u8}[])
            }
            frame "GrayC" {
              w532 = u8 255 ("Red")
              w533 = u8 0 ("Blue")
              n195 = for {
                N: 254 -> [_]
                tunnel: w534 -> [w538]
                tunnel: [w536] -> w530 mode=indexing
                i -> [w537]
                n196 = Bundle By Name(cluster=w538, "Red"=w537, "Green"=w537, "Blue"=w537) -> (w536:cluster{"Red":u8, "Green":u8, "Blue":u8})
              }
              n197 = Bundle By Name(cluster=w534, "Red"=w533, "Green"=w532, "Blue"=w533) -> (w531:cluster{"Red":u8, "Green":u8, "Blue":u8})
              n198 = Bundle By Name(cluster=w534, "Red"=w532, "Green"=w533, "Blue"=w533) -> (w529:cluster{"Red":u8, "Green":u8, "Blue":u8})
              n199 = Build Array (concatenate)(w531, w530, w529) -> (w528:cluster{"Red":u8, "Green":u8, "Blue":u8}[])
            }
            frame "GrayAB" {
              w546 = u8 255 ("Red")
              w547 = u8 0 ("Blue")
              n200 = Divide(x=150.0, y=253.0) -> (x/y=w539:dbl)
              n201 = for {
                N: 254 -> [_]
                tunnel: w548 -> [w557]
                tunnel: [w556] -> w544 mode=indexing
                tunnel: w539 -> [w554]
                i -> [w555]
                n202 = Multiply(x=w555, y=w554) -> (x*y=w553:dbl)
                n203 = To Unsigned Byte Integer(number=w553) -> (unsigned 8bit integer=w552:u8)
                n204 = Add(x=u8 75, y=w552) -> (x+y=w550:u8)
                n205 = Bundle By Name(cluster=w557, "Red"=w550, "Green"=w550, "Blue"=w550) -> (w556:cluster{"Red":u8, "Green":u8, "Blue":u8})
              }
              n206 = Bundle By Name(cluster=w548, "Red"=w547, "Green"=w546, "Blue"=w547) -> (w545:cluster{"Red":u8, "Green":u8, "Blue":u8})
              n207 = Bundle By Name(cluster=w548, "Red"=w546, "Green"=w547, "Blue"=w547) -> (w543:cluster{"Red":u8, "Green":u8, "Blue":u8})
              n208 = Build Array (concatenate)(w545, w544, w543) -> (w542:cluster{"Red":u8, "Green":u8, "Blue":u8}[])
            }
            frame "BGRN" {
              w567 = 64
              w560 = u8 255 ("Red")
              n209 = for {
                N: w567 -> [_]
                tunnel: w561 -> [w596]
                tunnel: [w590] -> w563 mode=indexing
                i -> [w592]
                n210 = Multiply(x=w592, y=4) -> (x*y=w593:i32)
                n211 = Bundle By Name(cluster=w596, "Red"=u8 0, "Green"=u8 0, "Blue"=w593) -> (w590:cluster{"Red":u8, "Green":u8, "Blue":u8})
              }
              n212 = for {
                N: w567 -> [_]
                tunnel: w561 -> [w589]
                tunnel: [w585] -> w564 mode=indexing
                i -> [w587]
                n213 = Multiply(x=w587, y=4) -> (x*y=w583:i32)
                n214 = Subtract(x=255, y=w583) -> (x-y=w584:i32)
                n215 = Bundle By Name(cluster=w589, "Red"=u8 0, "Green"=w583, "Blue"=w584) -> (w585:cluster{"Red":u8, "Green":u8, "Blue":u8})
              }
              n216 = for {
                N: w567 -> [_]
                tunnel: w561 -> [w581]
                tunnel: [w577] -> w565 mode=indexing
                i -> [w579]
                n217 = Multiply(x=w579, y=4) -> (x*y=w575:i32)
                n218 = Subtract(x=255, y=w575) -> (x-y=w576:i32)
                n219 = Bundle By Name(cluster=w581, "Blue"=u8 0 ("Red"), "Red"=w575, "Green"=w576) -> (w577:cluster{"Red":u8, "Green":u8, "Blue":u8})
              }
              n220 = for {
                N: 63 -> [_]
                tunnel: w561 -> [w573]
                tunnel: [w569] -> w562 mode=indexing
                i -> [w571]
                n221 = Multiply(x=w571, y=4) -> (x*y=w568:i32)
                n222 = Bundle By Name(cluster=w573, "Red"=u8 255, "Green"=w568, "Blue"=w568) -> (w569:cluster{"Red":u8, "Green":u8, "Blue":u8})
              }
              n223 = Bundle By Name(cluster=w561, "Red"=w560, "Green"=w560, "Blue"=w560) -> (w559:cluster{"Red":u8, "Green":u8, "Blue":u8})
              n224 = Build Array (concatenate)(w563, w564, w565, w562, w559) -> (w558:cluster{"Red":u8, "Green":u8, "Blue":u8}[])
            }
            frame "BGRAB" {
              w597 = 64
              w601 = u8 255 ("Red")
              n225 = for {
                N: 63 -> [_]
                tunnel: w598 -> [w638]
                tunnel: [w634] -> w603 mode=indexing
                i -> [w636]
                n226 = Increment(x=w636) -> (x+1=w631:i32)
                n227 = Multiply(x=w631, y=4) -> (x*y=w632:i32)
                n228 = Bundle By Name(cluster=w638, "Red"=u8 0, "Green"=w632, "Blue"=u8 255) -> (w634:cluster{"Red":u8, "Green":u8, "Blue":u8})
              }
              n229 = for {
                N: w597 -> [_]
                tunnel: w598 -> [w630]
                tunnel: [w626] -> w604 mode=indexing
                i -> [w628]
                w623 = 255 ("x")
                n230 = Multiply(x=w628, y=4) -> (x*y=w624:i32)
                n231 = Subtract(x=w623, y=w624) -> (x-y=w625:i32)
                n232 = Bundle By Name(cluster=w630, "Red"=u8 0, "Green"=w623, "Blue"=w625) -> (w626:cluster{"Red":u8, "Green":u8, "Blue":u8})
              }
              n233 = for {
                N: w597 -> [_]
                tunnel: w598 -> [w622]
                tunnel: [w618] -> w605 mode=indexing
                i -> [w620]
                n234 = Multiply(x=w620, y=4) -> (x*y=w616:i32)
                n235 = Bundle By Name(cluster=w622, "Blue"=u8 0 ("Red"), "Red"=w616, "Green"=255 ("x")) -> (w618:cluster{"Red":u8, "Green":u8, "Blue":u8})
              }
              n236 = for {
                N: 63 -> [_]
                tunnel: w598 -> [w615]
                tunnel: [w612] -> w602 mode=indexing
                i -> [w614]
                w609 = u8 255 ("Red")
                n237 = Multiply(x=w614, y=4) -> (x*y=w608:i32)
                n238 = Subtract(x=w609, y=w608) -> (x-y=w610:i32)
                n239 = Bundle By Name(cluster=w615, "Blue"=u8 0, "Red"=w609, "Green"=w610) -> (w612:cluster{"Red":u8, "Green":u8, "Blue":u8})
              }
              n240 = Bundle By Name(cluster=w598, "Red"=w601, "Green"=w601, "Blue"=w601) -> (w600:cluster{"Red":u8, "Green":u8, "Blue":u8})
              n241 = Build Array (concatenate)(w598, w603, w604, w605, w602, w600) -> (w599:cluster{"Red":u8, "Green":u8, "Blue":u8}[])
            }
            frame "BGRN+-" {
              w650 = 32
              w643 = u8 255 ("Red")
              n242 = for {
                N: w650 -> [_]
                tunnel: w644 -> [w679]
                tunnel: [w673] -> w646 mode=indexing
                i -> [w675]
                n243 = Multiply(x=w675, y=8) -> (x*y=w676:i32)
                n244 = Bundle By Name(cluster=w679, "Red"=u8 0, "Green"=u8 0, "Blue"=w676) -> (w673:cluster{"Red":u8, "Green":u8, "Blue":u8})
              }
              n245 = for {
                N: w650 -> [_]
                tunnel: w644 -> [w672]
                tunnel: [w668] -> w647 mode=indexing
                i -> [w670]
                n246 = Multiply(x=w670, y=8) -> (x*y=w666:i32)
                n247 = Subtract(x=255, y=w666) -> (x-y=w667:i32)
                n248 = Bundle By Name(cluster=w672, "Red"=u8 0, "Green"=w666, "Blue"=w667) -> (w668:cluster{"Red":u8, "Green":u8, "Blue":u8})
              }
              n249 = for {
                N: w650 -> [_]
                tunnel: w644 -> [w664]
                tunnel: [w660] -> w648 mode=indexing
                i -> [w662]
                n250 = Multiply(x=w662, y=8) -> (x*y=w658:i32)
                n251 = Subtract(x=255, y=w658) -> (x-y=w659:i32)
                n252 = Bundle By Name(cluster=w664, "Blue"=u8 0 ("Red"), "Red"=w658, "Green"=w659) -> (w660:cluster{"Red":u8, "Green":u8, "Blue":u8})
              }
              n253 = for {
                N: 31 -> [_]
                tunnel: w644 -> [w656]
                tunnel: [w652] -> w645 mode=indexing
                i -> [w654]
                n254 = Multiply(x=w654, y=8) -> (x*y=w651:i32)
                n255 = Bundle By Name(cluster=w656, "Red"=u8 255, "Green"=w651, "Blue"=w651) -> (w652:cluster{"Red":u8, "Green":u8, "Blue":u8})
              }
              n256 = Bundle By Name(cluster=w644, "Red"=w643, "Green"=w643, "Blue"=w643) -> (w642:cluster{"Red":u8, "Green":u8, "Blue":u8})
              n257 = Build Array (concatenate)(w646, w647, w648, w645, w642) -> (w641:cluster{"Red":u8, "Green":u8, "Blue":u8}[])
              n258 = Reverse 1D Array(array=w641) -> (reversed array=w640:cluster{"Red":u8, "Green":u8, "Blue":u8}[])
              n259 = Build Array (concatenate)(w640, w641) -> (w639:cluster{"Red":u8, "Green":u8, "Blue":u8}[])
            }
            frame "BGRL" {
              w680 = 32
              w684 = u8 255 ("Red")
              n260 = for {
                N: w680 -> [_]
                tunnel: w685 -> [w719]
                tunnel: [w713] -> w687 mode=indexing
                i -> [w715]
                n261 = Multiply(x=w715, y=8) -> (x*y=w716:i32)
                n262 = Bundle By Name(cluster=w719, "Red"=u8 0, "Green"=u8 0, "Blue"=w716) -> (w713:cluster{"Red":u8, "Green":u8, "Blue":u8})
              }
              n263 = for {
                N: w680 -> [_]
                tunnel: w685 -> [w712]
                tunnel: [w708] -> w688 mode=indexing
                i -> [w710]
                n264 = Multiply(x=w710, y=8) -> (x*y=w706:i32)
                n265 = Subtract(x=255, y=w706) -> (x-y=w707:i32)
                n266 = Bundle By Name(cluster=w712, "Red"=u8 0, "Green"=w706, "Blue"=w707) -> (w708:cluster{"Red":u8, "Green":u8, "Blue":u8})
              }
              n267 = for {
                N: 64 -> [_]
                tunnel: w685 -> [w704]
                tunnel: [w700] -> w689 mode=indexing
                i -> [w702]
                n268 = Multiply(x=w702, y=4) -> (x*y=w698:i32)
                n269 = Subtract(x=255, y=w698) -> (x-y=w699:i32)
                n270 = Bundle By Name(cluster=w704, "Blue"=u8 0 ("Red"), "Red"=w698, "Green"=w699) -> (w700:cluster{"Red":u8, "Green":u8, "Blue":u8})
              }
              n271 = for {
                N: 127 -> [_]
                tunnel: w685 -> [w696]
                tunnel: [w692] -> w686 mode=indexing
                i -> [w694]
                n272 = Multiply(x=w694, y=2) -> (x*y=w691:i32)
                n273 = Bundle By Name(cluster=w696, "Red"=u8 255, "Green"=w691, "Blue"=w691) -> (w692:cluster{"Red":u8, "Green":u8, "Blue":u8})
              }
              n274 = Bundle By Name(cluster=w685, "Red"=w684, "Green"=w684, "Blue"=w684) -> (w683:cluster{"Red":u8, "Green":u8, "Blue":u8})
              n275 = Build Array (concatenate)(w687, w688, w689, w686, w683) -> (w682:cluster{"Red":u8, "Green":u8, "Blue":u8}[])
            }
            frame "BGRL+-" {
              w723 = 16
              w726 = u8 255 ("Red")
              n276 = for {
                N: w723 -> [_]
                tunnel: w727 -> [w761]
                tunnel: [w755] -> w729 mode=indexing
                i -> [w757]
                n277 = Multiply(x=w757, y=16) -> (x*y=w758:i32)
                n278 = Bundle By Name(cluster=w761, "Red"=u8 0, "Green"=u8 0, "Blue"=w758) -> (w755:cluster{"Red":u8, "Green":u8, "Blue":u8})
              }
              n279 = for {
                N: w723 -> [_]
                tunnel: w727 -> [w754]
                tunnel: [w750] -> w730 mode=indexing
                i -> [w752]
                n280 = Multiply(x=w752, y=16) -> (x*y=w748:i32)
                n281 = Subtract(x=255, y=w748) -> (x-y=w749:i32)
                n282 = Bundle By Name(cluster=w754, "Red"=u8 0, "Green"=w748, "Blue"=w749) -> (w750:cluster{"Red":u8, "Green":u8, "Blue":u8})
              }
              n283 = for {
                N: 32 -> [_]
                tunnel: w727 -> [w746]
                tunnel: [w742] -> w731 mode=indexing
                i -> [w744]
                n284 = Multiply(x=w744, y=8) -> (x*y=w740:i32)
                n285 = Subtract(x=255, y=w740) -> (x-y=w741:i32)
                n286 = Bundle By Name(cluster=w746, "Blue"=u8 0 ("Red"), "Red"=w740, "Green"=w741) -> (w742:cluster{"Red":u8, "Green":u8, "Blue":u8})
              }
              n287 = for {
                N: 63 -> [_]
                tunnel: w727 -> [w738]
                tunnel: [w734] -> w728 mode=indexing
                i -> [w736]
                n288 = Multiply(x=w736, y=4) -> (x*y=w733:i32)
                n289 = Bundle By Name(cluster=w738, "Red"=u8 255, "Green"=w733, "Blue"=w733) -> (w734:cluster{"Red":u8, "Green":u8, "Blue":u8})
              }
              n290 = Bundle By Name(cluster=w727, "Red"=w726, "Green"=w726, "Blue"=w726) -> (w725:cluster{"Red":u8, "Green":u8, "Blue":u8})
              n291 = Build Array (concatenate)(w729, w730, w731, w728, w725) -> (w722:cluster{"Red":u8, "Green":u8, "Blue":u8}[])
              n292 = Reverse 1D Array(array=w722) -> (reversed array=w721:cluster{"Red":u8, "Green":u8, "Blue":u8}[])
              n293 = Build Array (concatenate)(w721, w722) -> (w720:cluster{"Red":u8, "Green":u8, "Blue":u8}[])
            }
            frame "BGRH" {
              w767 = u8 255 ("Red")
              n294 = for {
                N: 128 -> [_]
                tunnel: w768 -> [w802]
                tunnel: [w796] -> w770 mode=indexing
                i -> [w798]
                n295 = Multiply(x=w798, y=2) -> (x*y=w799:i32)
                n296 = Bundle By Name(cluster=w802, "Red"=u8 0, "Green"=u8 0, "Blue"=w799) -> (w796:cluster{"Red":u8, "Green":u8, "Blue":u8})
              }
              n297 = for {
                N: 64 -> [_]
                tunnel: w768 -> [w795]
                tunnel: [w791] -> w771 mode=indexing
                i -> [w793]
                n298 = Multiply(x=w793, y=4) -> (x*y=w789:i32)
                n299 = Subtract(x=255, y=w789) -> (x-y=w790:i32)
                n300 = Bundle By Name(cluster=w795, "Red"=u8 0, "Green"=w789, "Blue"=w790) -> (w791:cluster{"Red":u8, "Green":u8, "Blue":u8})
              }
              n301 = for {
                N: 32 -> [_]
                tunnel: w768 -> [w787]
                tunnel: [w783] -> w772 mode=indexing
                i -> [w785]
                n302 = Multiply(x=w785, y=8) -> (x*y=w781:i32)
                n303 = Subtract(x=255, y=w781) -> (x-y=w782:i32)
                n304 = Bundle By Name(cluster=w787, "Blue"=u8 0 ("Red"), "Red"=w781, "Green"=w782) -> (w783:cluster{"Red":u8, "Green":u8, "Blue":u8})
              }
              n305 = for {
                N: 31 -> [_]
                tunnel: w768 -> [w779]
                tunnel: [w775] -> w769 mode=indexing
                i -> [w777]
                n306 = Multiply(x=w777, y=8) -> (x*y=w774:i32)
                n307 = Bundle By Name(cluster=w779, "Red"=u8 255, "Green"=w774, "Blue"=w774) -> (w775:cluster{"Red":u8, "Green":u8, "Blue":u8})
              }
              n308 = Bundle By Name(cluster=w768, "Red"=w767, "Green"=w767, "Blue"=w767) -> (w766:cluster{"Red":u8, "Green":u8, "Blue":u8})
              n309 = Build Array (concatenate)(w770, w771, w772, w769, w766) -> (w765:cluster{"Red":u8, "Green":u8, "Blue":u8}[])
            }
            frame "BGRH+-" {
              w810 = u8 255 ("Red")
              n310 = for {
                N: 64 -> [_]
                tunnel: w811 -> [w845]
                tunnel: [w839] -> w813 mode=indexing
                i -> [w841]
                n311 = Multiply(x=w841, y=4) -> (x*y=w842:i32)
                n312 = Bundle By Name(cluster=w845, "Red"=u8 0, "Green"=u8 0, "Blue"=w842) -> (w839:cluster{"Red":u8, "Green":u8, "Blue":u8})
              }
              n313 = for {
                N: 32 -> [_]
                tunnel: w811 -> [w838]
                tunnel: [w834] -> w814 mode=indexing
                i -> [w836]
                n314 = Multiply(x=w836, y=8) -> (x*y=w832:i32)
                n315 = Subtract(x=255, y=w832) -> (x-y=w833:i32)
                n316 = Bundle By Name(cluster=w838, "Red"=u8 0, "Green"=w832, "Blue"=w833) -> (w834:cluster{"Red":u8, "Green":u8, "Blue":u8})
              }
              n317 = for {
                N: 16 -> [_]
                tunnel: w811 -> [w830]
                tunnel: [w826] -> w815 mode=indexing
                i -> [w828]
                n318 = Multiply(x=w828, y=16) -> (x*y=w824:i32)
                n319 = Subtract(x=255, y=w824) -> (x-y=w825:i32)
                n320 = Bundle By Name(cluster=w830, "Blue"=u8 0 ("Red"), "Red"=w824, "Green"=w825) -> (w826:cluster{"Red":u8, "Green":u8, "Blue":u8})
              }
              n321 = for {
                N: 15 -> [_]
                tunnel: w811 -> [w822]
                tunnel: [w818] -> w812 mode=indexing
                i -> [w820]
                n322 = Multiply(x=w820, y=16) -> (x*y=w817:i32)
                n323 = Bundle By Name(cluster=w822, "Red"=u8 255, "Green"=w817, "Blue"=w817) -> (w818:cluster{"Red":u8, "Green":u8, "Blue":u8})
              }
              n324 = Bundle By Name(cluster=w811, "Red"=w810, "Green"=w810, "Blue"=w810) -> (w809:cluster{"Red":u8, "Green":u8, "Blue":u8})
              n325 = Build Array (concatenate)(w813, w814, w815, w812, w809) -> (w805:cluster{"Red":u8, "Green":u8, "Blue":u8}[])
              n326 = Reverse 1D Array(array=w805) -> (reversed array=w804:cluster{"Red":u8, "Green":u8, "Blue":u8}[])
              n327 = Build Array (concatenate)(w804, w805) -> (w803:cluster{"Red":u8, "Green":u8, "Blue":u8}[])
            }
            frame "Phase" {
              w847 = 85
              n328 = for {
                N: 43 -> [_]
                tunnel: w849 -> [w887]
                tunnel: [w884] -> w851 mode=indexing
                i -> [w886]
                w880 = 127 ("x")
                n329 = Multiply(x=w886, y=3) -> (x*y=w882:i32)
                n330 = Subtract(x=w880, y=w882) -> (x-y=w881:i32)
                n331 = Add(x=w882, y=w880) -> (x+y=w879:i32)
                n332 = Bundle By Name(cluster=w887, "Red"=w881, "Green"=u8 0 ("Red"), "Blue"=w879) -> (w884:cluster{"Red":u8, "Green":u8, "Blue":u8})
              }
              n333 = for {
                N: w847 -> [_]
                tunnel: w849 -> [w878]
                tunnel: [w874] -> w852 mode=indexing
                i -> [w876]
                n334 = Multiply(x=w876, y=3) -> (x*y=w872:i32)
                n335 = Subtract(x=255, y=w872) -> (x-y=w873:i32)
                n336 = Bundle By Name(cluster=w878, "Red"=u8 0, "Green"=w872, "Blue"=w873) -> (w874:cluster{"Red":u8, "Green":u8, "Blue":u8})
              }
              n337 = for {
                N: w847 -> [_]
                tunnel: w849 -> [w870]
                tunnel: [w866] -> w853 mode=indexing
                i -> [w868]
                n338 = Multiply(x=w868, y=3) -> (x*y=w864:i32)
                n339 = Subtract(x=255, y=w864) -> (x-y=w865:i32)
                n340 = Bundle By Name(cluster=w870, "Blue"=u8 0 ("Red"), "Red"=w864, "Green"=w865) -> (w866:cluster{"Red":u8, "Green":u8, "Blue":u8})
              }
              n341 = for {
                N: 43 -> [_]
                tunnel: w849 -> [w862]
                tunnel: [w859] -> w850 mode=indexing
                i -> [w861]
                n342 = Multiply(x=w861, y=3) -> (x*y=w855:i32)
                n343 = Subtract(x=255 ("Red"), y=w855) -> (x-y=w857:i32)
                n344 = Bundle By Name(cluster=w862, "Red"=w857, "Green"=u8 0 ("Blue"), "Blue"=w855) -> (w859:cluster{"Red":u8, "Green":u8, "Blue":u8})
              }
              n345 = Build Array (concatenate)(w851, w852, w853, w850) -> (w848:cluster{"Red":u8, "Green":u8, "Blue":u8}[])
            }
            frame "BWR" {
              w888 = 85
              w892 = u8 255 ("Red")
              n346 = for {
                N: 86 ("Dimension Size") -> [_]
                tunnel: w894 -> [w903]
                tunnel: [w900] -> w896 mode=indexing
                i -> [w902]
                w897 = 255 ("x")
                n347 = Multiply(x=w902, y=3) -> (x*y=w899:i32)
                n348 = Subtract(x=w897, y=w899) -> (x-y=w898:i32)
                n349 = Bundle By Name(cluster=w903, "Blue"=w898, "Red"=w897, "Green"=w898) -> (w900:cluster{"Red":u8, "Green":u8, "Blue":u8})
              }
              n350 = for {
                N: w888 -> [_]
                tunnel: w894 -> [w909]
                tunnel: [w906] -> w895 mode=indexing
                i -> [w908]
                n351 = Multiply(x=w908, y=3) -> (x*y=w904:i32)
                n352 = Bundle By Name(cluster=w909, "Red"=w904, "Green"=w904, "Blue"=u8 255) -> (w906:cluster{"Red":u8, "Green":u8, "Blue":u8})
              }
              n353 = Bundle By Name(cluster=w894, "Red"=w892, "Green"=w892, "Blue"=w892) -> (w891:cluster{"Red":u8, "Green":u8, "Blue":u8})
              n354 = Initialize Array(w891, w888) -> (w890:cluster{"Red":u8, "Green":u8, "Blue":u8}[])
              n355 = Build Array (concatenate)(w895, w890, w896) -> (w893:cluster{"Red":u8, "Green":u8, "Blue":u8}[])
            }
            frame "BR" {
              w912 = 128
              n356 = for {
                N: w912 -> [_]
                tunnel: w913 -> [w929]
                tunnel: [w928] -> w915 mode=indexing
                i -> [w924]
                n357 = Quotient & Remainder(x=w924, y=2) -> (floor(x/y)=w925:i32)  [unwired: 1 out]
                n358 = Add(x=w924, y=w925) -> (x+y=w923:i32)
                n359 = Bundle By Name(cluster=w929, "Red"=w923, "Green"=w923, "Blue"=u8 255) -> (w928:cluster{"Red":u8, "Green":u8, "Blue":u8})
              }
              n360 = for {
                N: w912 -> [_]
                tunnel: w913 -> [w922]
                tunnel: [w921] -> w911 mode=indexing
                i -> [w918]
                n361 = Quotient & Remainder(x=w918, y=2) -> (floor(x/y)=w919:i32)  [unwired: 1 out]
                n362 = Add(x=w918, y=w919) -> (x+y=w917:i32)
                n363 = Bundle By Name(cluster=w922, "Red"=u8 255 ("Blue"), "Green"=w917, "Blue"=w917) -> (w921:cluster{"Red":u8, "Green":u8, "Blue":u8})
              }
              n364 = Reverse 1D Array(array=w911) -> (reversed array=w910:cluster{"Red":u8, "Green":u8, "Blue":u8}[])
              n365 = Build Array (concatenate)(w915, w910) -> (w914:cluster{"Red":u8, "Green":u8, "Blue":u8}[])
            }
            frame "BkW" {
              w931 = 127 ("dimension size")
              w936 = u8 255 ("Red")
              w937 = u8 0 ("Blue")
              n366 = Bundle By Name(cluster=w938, "Red"=w937, "Green"=w937, "Blue"=w936) -> (w935:cluster{"Red":u8, "Green":u8, "Blue":u8})
              n367 = Bundle By Name(cluster=w938, "Red"=w937, "Green"=w937, "Blue"=w937) -> (w934:cluster{"Red":u8, "Green":u8, "Blue":u8})
              n368 = Bundle By Name(cluster=w938, "Red"=w936, "Green"=w936, "Blue"=w936) -> (w932:cluster{"Red":u8, "Green":u8, "Blue":u8})
              n369 = Initialize Array(w934, w931) -> (w933:cluster{"Red":u8, "Green":u8, "Blue":u8}[])
              n370 = Initialize Array(w932, w931) -> (w930:cluster{"Red":u8, "Green":u8, "Blue":u8}[])
              n371 = Build Array (concatenate)(w935, w933, w930, w935) -> (w939:cluster{"Red":u8, "Green":u8, "Blue":u8}[])
            }
          }
          n372 = Array Size(array=w395) -> (size(s)=w394:i32)
          n373 = Subtract(x=w398, y=w397) -> (x-y=w396:dbl)
          n374 = Decrement(x=w394) -> (x-1=w393:i32)
          n375 = Divide(x=w396, y=w393) -> (x/y=w392:dbl)
          n376 = for {
            tunnel: w395 -> [w414] mode=indexing
            tunnel: w397 -> [w406]
            tunnel: w392 -> [w405]
            tunnel: [w401] -> w391 mode=indexing
            i -> [w404]
            n377 = Unbundle By Name(w414) -> ("Red"=w411:u8, "Green"=w413:u8, "Blue"=w412:u8)
            n378 = Multiply(x=w405, y=w404) -> (x*y=w403:dbl)
            n379 = Join Numbers(hi=u8 0, lo=w411) -> ((hi.lo)=w409:u16)
            n380 = Join Numbers(hi=w413, lo=w412) -> ((hi.lo)=w408:u16)
            n381 = Join Numbers(hi=w409, lo=w408) -> ((hi.lo)=w402:u32)
            n382 = Add(x=w406, y=w403) -> (x+y=w407:dbl)
            n383 = Bundle(w407, w402) -> (w401:cluster{dbl, u32})  [unwired: 1 out]
          }
        }
      }
      n384 = Array Size(array=w11) -> (size(s)=w19:i32)
      n385 = Decrement(x=w19) -> (x-1=w18:i32)
      n386 = Index Array(array=w11, index #1=0 ("index"), index #2=w18) -> (element #1=w17:cluster{"Max":dbl, "Color":u32}, element #2=w14:cluster{"Max":dbl, "Color":u32})
      n387 = Unbundle By Name(w14) -> ("Color"=w15:u32)
      n388 = Unbundle By Name(w17) -> ("Color"=w16:u32)
      n389 = Not A Number/Path/Refnum?(number/path/refnum=w13) -> (NaN/Path/Refnum?=w12:bool)
      n390 = case shown="False" w12 {
        tunnel: [w36 w77] -> w23
        tunnel: w22 -> [w30 w76]
        tunnel: [w35 w76] -> w21
        tunnel: w16 -> [w34 _]
        tunnel: w15 -> [w33 _]
        tunnel: w11 -> [w32 _]
        tunnel: w13 -> [w31 w77]
        frame False {
          n391 = property on="Property Node" class="GObj"(reference=w31, error in=w30) -> (reference out=w27:refnum<vi>, error out=w28:errorcluster, "Class ID"=w29:u32)
          n392 = case shown="43" w29 {
            tunnel: [w46 w56 w58 w75] -> w36
            tunnel: [w45 w55 w59 w74] -> w35
            tunnel: w34 -> [w44 w54 _ w73]
            tunnel: w33 -> [w43 w53 _ w72]
            tunnel: w32 -> [w42 w52 _ w71]
            tunnel: w28 -> [w41 w51 _ w70]
            tunnel: w27 -> [w40 w50 w58 w69]
            frame 26 {
              w38 = refnum<vi> refnum  # IntensityGraph
              n393 = To More Specific Class(target class=w38, reference=w40, error in=w41) -> (specific class reference=w37:refnum<vi>, error out=w39:errorcluster)
              n394 = property on="Property Node" class="IntGraph"(reference=w37, error in=w39, "Z Scale.Low Color"=w44, "Z Scale.High Color"=w43, "Z Scale.Marker Values[]"=w42) -> (reference out=w46:refnum<vi>, error out=w45:errorcluster)
            }
            frame 25 {
              w48 = refnum<vi> refnum  # IntensityChart
              n395 = To More Specific Class(target class=w48, reference=w50, error in=w51) -> (specific class reference=w47:refnum<vi>, error out=w49:errorcluster)
              n396 = property on="Property Node" class="IntChart"(reference=w47, error in=w49, "Z Scale.Low Color"=w54, "Z Scale.High Color"=w53, "Z Scale.Marker Values[]"=w52) -> (reference out=w56:refnum<vi>, error out=w55:errorcluster)
            }
            frame Default {
              n397 = Call Chain() -> (call chain=w65:string[])
              n398 = Array To Spreadsheet String(delimiter (Tab)="->", array=w65, 3:"%s" ("format string")) -> (spreadsheet string=w62:string)
              n399 = Format Into String(format string="%s\nReference must be Intensity Graph or Color Scale.", w62) -> (resulting string=w57:string)  [unwired: 2 in, 1 out]
              n400 = Bundle By Name(cluster=errorcluster {"status"=TRUE, "code"=1, "source"=""} ("error out"), "source"=w57) -> (w59:errorcluster)
            }
            frame 43 {
              w67 = refnum<vi> refnum  # ColorGraphScale
              n401 = To More Specific Class(target class=w67, reference=w69, error in=w70) -> (specific class reference=w66:refnum<vi>, error out=w68:errorcluster)
              n402 = property on="Property Node" class="ColGrphScl"(reference=w66, error in=w68, "Low Color"=w73, "High Color"=w72, "Marker Values[]"=w71) -> (reference out=w75:refnum<vi>, error out=w74:errorcluster)
            }
          }
        }
        frame True {
        }
      }
    }
    frame Error {
    }
  }
  "ValueScale" <- w4
  "error out" <- w5
  "Ref (Duplicate)" <- w6
